vi "Impedance Equivalent Circuit Identifier.vi"(8 "error in (no error)":errorcluster, 9 "type in original":T1=enum."Rs-Xs", 10 "type in by string":string, 11 "type in":T1=enum."Rs-Xs") -> (0 "error out":errorcluster, 2 "type info":T2, 3 "type out":T1=enum."Rs-Xs")   [LabVIEW 2020]
doc: "Impedance equivalent circuit connection convertor: identify equ connection from string or direct type in and return type id and type info."
uses:
  Impedance Equivalent Circuit.ctl
  Impedance Equivalent Circuit Type Info.ctl
  <vilib>/Utility/error.llb/Error Cluster From Error Code.vi
  <vilib>/ErrorRing/Error Ring.xnode
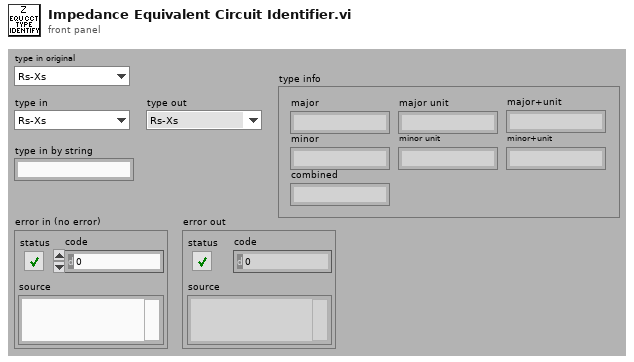
[diagram p1: front panel]
types:
  T1 = typedef "Impedance Equivalent Circuit.ctl" = enum16{"Keep original", "Rs-Xs", "Gp-Bp", "Z-phid", "Z-phir", "Y-phid", "Y-phir", "Cp-D", "Cp-Q", "Cp-Rp", "Cp-Gp", "Cs-D", "Cs-Q", "Cs-Rs", "Ls-Rs", "Ls-Q", "Rs-Tau"}
  T2 = typedef "Impedance Equivalent Circuit Type Info.ctl" = cluster{"major":string, "major unit":string, "minor":string, "minor unit":string, "combined":string, "major+unit":string, "minor+unit":string}
  T3 = cluster{"major":string, "minor":string, "major unit":string, "minor unit":string}[]
  T4 = cluster{"major":string, "minor":string, "major unit":string, "minor unit":string}
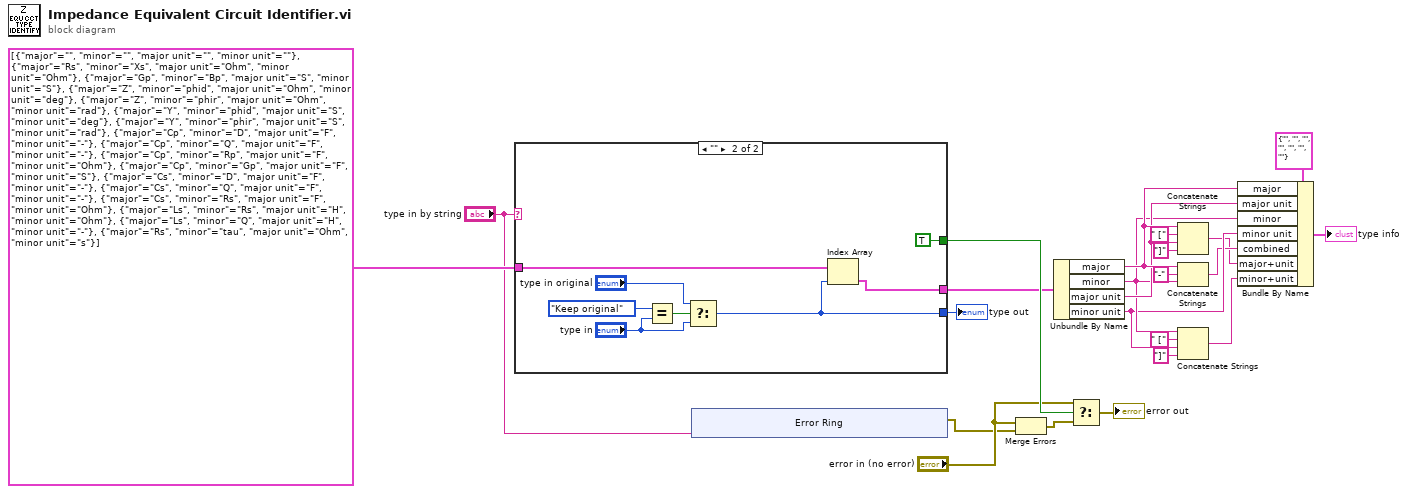
[diagram p0: block diagram]
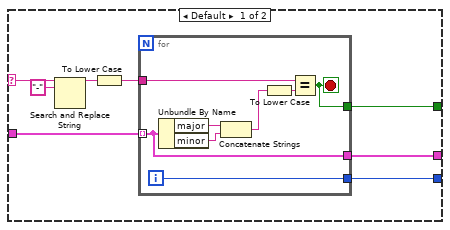
[diagram p2: hidden frame]
diagram:
  n1 = case shown="\"\"" "type in by string" {
    selector: "type in by string" -> [w29 _]
    tunnel: T3 [{"major"="", "minor"="", "major unit"="", "minor unit"=""}, {"major"="Rs", "minor"="Xs", "major unit"="Ohm", "minor unit"="Ohm"}, {"major"="Gp", "minor"="Bp", "major unit"="S", "minor unit"="S"}, {"major"="Z", "minor"="phid", "major unit"="Ohm", "minor unit"="deg"}, {"major"="Z", "minor"="phir", "major unit"="Ohm", "minor unit"="rad"}, {"major"="Y", "minor"="phid", "major unit"="S", "minor unit"="deg"}, {"major"="Y", "minor"="phir", "major unit"="S", "minor unit"="rad"}, {"major"="Cp", "minor"="D", "major unit"="F", "minor unit"="-"}, {"major"="Cp", "minor"="Q", "major unit"="F", "minor unit"="-"}, {"major"="Cp", "minor"="Rp", "major unit"="F", "minor unit"="Ohm"}, {"major"="Cp", "minor"="Gp", "major unit"="F", "minor unit"="S"}, {"major"="Cs", "minor"="D", "major unit"="F", "minor unit"="-"}, {"major"="Cs", "minor"="Q", "major unit"="F", "minor unit"="-"}, {"major"="Cs", "minor"="Rs", "major unit"="F", "minor unit"="Ohm"}, {"major"="Ls", "minor"="Rs", "major unit"="H", "minor unit"="Ohm"}, {"major"="Ls", "minor"="Q", "major unit"="H", "minor unit"="-"}, {"major"="Rs", "minor"="tau", "major unit"="Ohm", "minor unit"="s"}] -> [w28 w47]
    tunnel: [w27 TRUE] -> w20
    tunnel: [w25 w46] -> w15
    tunnel: [w24 w40] -> w22
    frame Default {
      n2 = Search and Replace String(input string=w29, search string="-") -> (result string=w30:string)  [unwired: 6 in, 3 out]
      n3 = To Lower Case(string=w30) -> (all lower case string=w26:string)
      n4 = for {
        tunnel: w26 -> [w39]
        tunnel: w28 -> [w35] mode=indexing
        tunnel: [w35] -> w25
        tunnel: [w34] -> w27
        tunnel: [w32] -> w24
        i -> [w32]
        stop <- w34 stop-if-true
        n5 = Unbundle By Name(w35) -> ("major"=w38:string, "minor"=w37:string)
        n6 = Concatenate Strings(w38, w37) -> (w36:string)
        n7 = To Lower Case(string=w36) -> (all lower case string=w33:string)
        n8 = Equal?(x=w39, y=w33) -> (x = y?=w34:bool)
      }
    }
    frame "" {
      n9 = Equal?(x=Impedance_Equivalent_Circuit."Keep original", y="type in") -> (x = y?=w43:bool)
      n10 = Select(t="type in original", s=w43, f="type in") -> (s? t:f=w40:T1)
      n11 = Index Array(array=w47, index=w40) -> (element=w46:T4)
    }
  }
  "type out" <- w22
  n12 = xnode "Error Ring"("parameter 0"="type in by string") -> ("error out"=w18:errorcluster)
  n13 = Merge Errors("error in (no error)", w18) -> (w17:errorcluster)
  n14 = Unbundle By Name(w15) -> ("major"=w8:string, "minor"=w6:string, "major unit"=w7:string, "minor unit"=w5:string)
  n15 = Select(t="error in (no error)", s=w20, f=w17) -> (s? t:f=→"error out":errorcluster)
  n16 = Concatenate Strings(w8, " [" ("string"), w7, "]" ("string")) -> (w3:string)
  n17 = Concatenate Strings(w8, "-" ("string"), w6) -> (w4:string)
  n18 = Concatenate Strings(w6, " [" ("string"), w5, "]" ("string")) -> (w2:string)
  n19 = Bundle By Name(cluster=T2 {"major"="", "major unit"="", "minor"="", "minor unit"="", "combined"="", "major+unit"="", "minor+unit"=""} ("type info"), "major"=w8, "major unit"=w7, "minor"=w6, "minor unit"=w5, "combined"=w4, "major+unit"=w3, "minor+unit"=w2) -> (→"type info":T2)
